vi "icListen 3 Reset.vi"() -> ()   [LabVIEW 2020, in "PAM Library.lvlib"]
uses:
  PAM Library.lvlib
panel:
  in  "icListen 3 Reset":bool
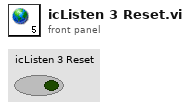
[diagram p1: front panel]
diagram:
